vi "Motor Controller two-parameter optimisation.vi"(0 "Settling time (ms)":u32=5000, 1 "Data rate (Hz)":u8(ring)=21 items=["1", "2", "4", "5", "8", "10", "16", "20", "25", "32", "40", "50", "64", "80", "100", "125", "160", "200", "250", "320", "400", "500", "625", "800", "1000"], 2 "N samples":i32=5000, 3 "Kp_start":dbl=9.999999747378752e-05 format="%#_6f", 4 "Kp_end":dbl=0.002 format="%#_6f", 5 "N_points_Kp":i32=30 min=1, 6 "RPM":sgl=600.0 format="%#_6f", 7 "Ti_start (s)":dbl=0.005 format="%#_6f", 8 "COM port":refnum<visa-resource-name>, 9 "Ti_end (s)":dbl=1.0 format="%#_6f", 11 "N_points_Ti":i32=30 min=1) -> (10 "Frm errs":u32, 12 "Chk errs":u32, 14 "Kp (/rpm)":string, 15 "Ti (s)":string, 16 "RPM std. dev. (/min)":string, 17 "Im mean (A)":string, 18 "Im std. dev. (A)":string, 19 "Error out":errorcluster)   [LabVIEW 2020]
uses:
  <vilib>/Math Plots/3D Math Plots/3D Surface/3D Surface XCtrl/3D Surface.xctl
  ctls/CTRL_PID_params.ctl
  <vilib>/Math Plots/3D Math Plots/3D Surface/3D Surface Datatype/Public/Plot Helper (Vector).vi
  <vilib>/Analysis/NI_AALBase.lvlib
  <vilib>/Math Plots/3D Math Plots/3D Surface/3D Surface Datatype/3D Surface Datatype.lvclass
panel:
  out "Ti loop":i32
  out "Kp loop":i32
  in  "Format string":string="%.6e"
  out "Stats plots":refnum<class "3D Plot Datatype.lvclass">[](xcontrol)
  in  "Stop":bool
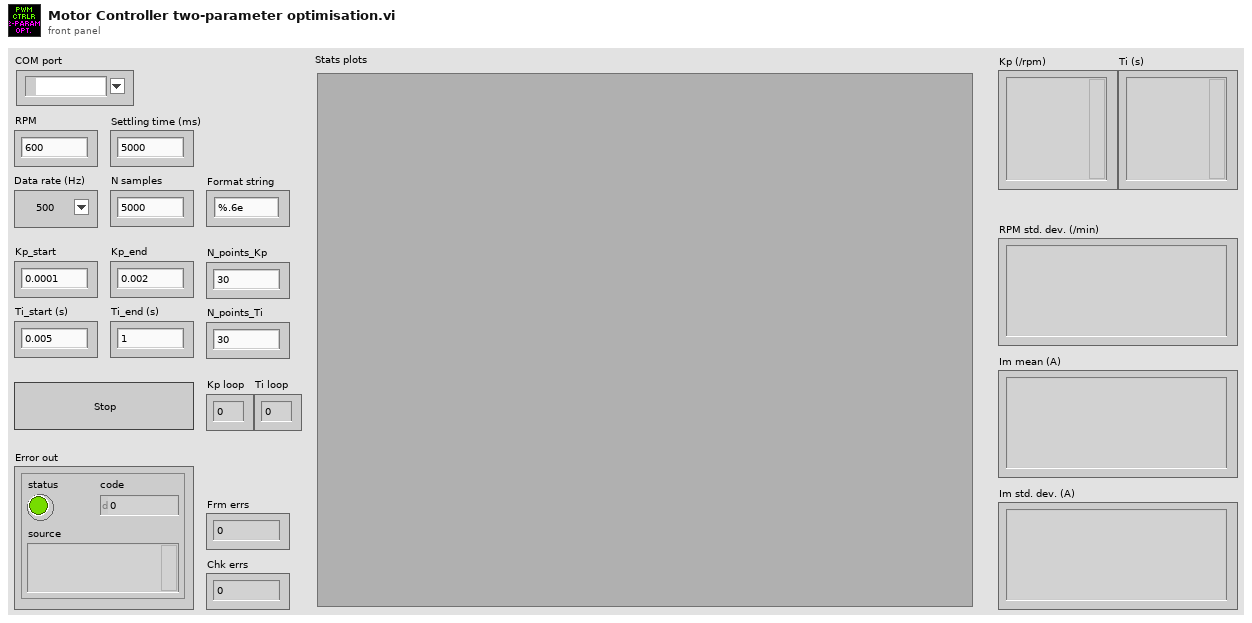
[diagram p1: front panel]
types:
  T1 = typedef "CTRL_EEPROM.ctl" = cluster{"N bits":u8, "dt (s)":sgl, "Kp (/rpm)":sgl, "Ti (s)":sgl, "Td (s)":sgl, "N bits_soft":u8, "dt_soft (s)":sgl, "Kp_soft (/rpm)":sgl, "Ti_soft (s)":sgl, "Td_soft (s)":sgl, "Encoder counting edges":u8, "Encoder PPR":u16, "Final drive ratio (X:1)":sgl, "Current zero offset (A)":sgl, "RS-485 address":u8, "RS-485 baud rate":u32, "Data output period (us)":u32, "RPM setpoint":sgl, "USB streaming enabled":bool, "Operating mode":u8, "Running mode":u8, "EEPROM CRC-16":u16}
  T2 = typedef "CTRL_PID_params.ctl" = cluster{"N bits":u8, "dt (s)":sgl, "Kp (/rpm)":sgl, "Ti (s)":sgl, "Td (s)":sgl}
  T3 = typedef "CTRL_Data_Out.ctl" = cluster{"RPM (/min)":sgl, "I_motor (A)":sgl, "V_photo (V)":sgl, "Duty (-1...1)":sgl}
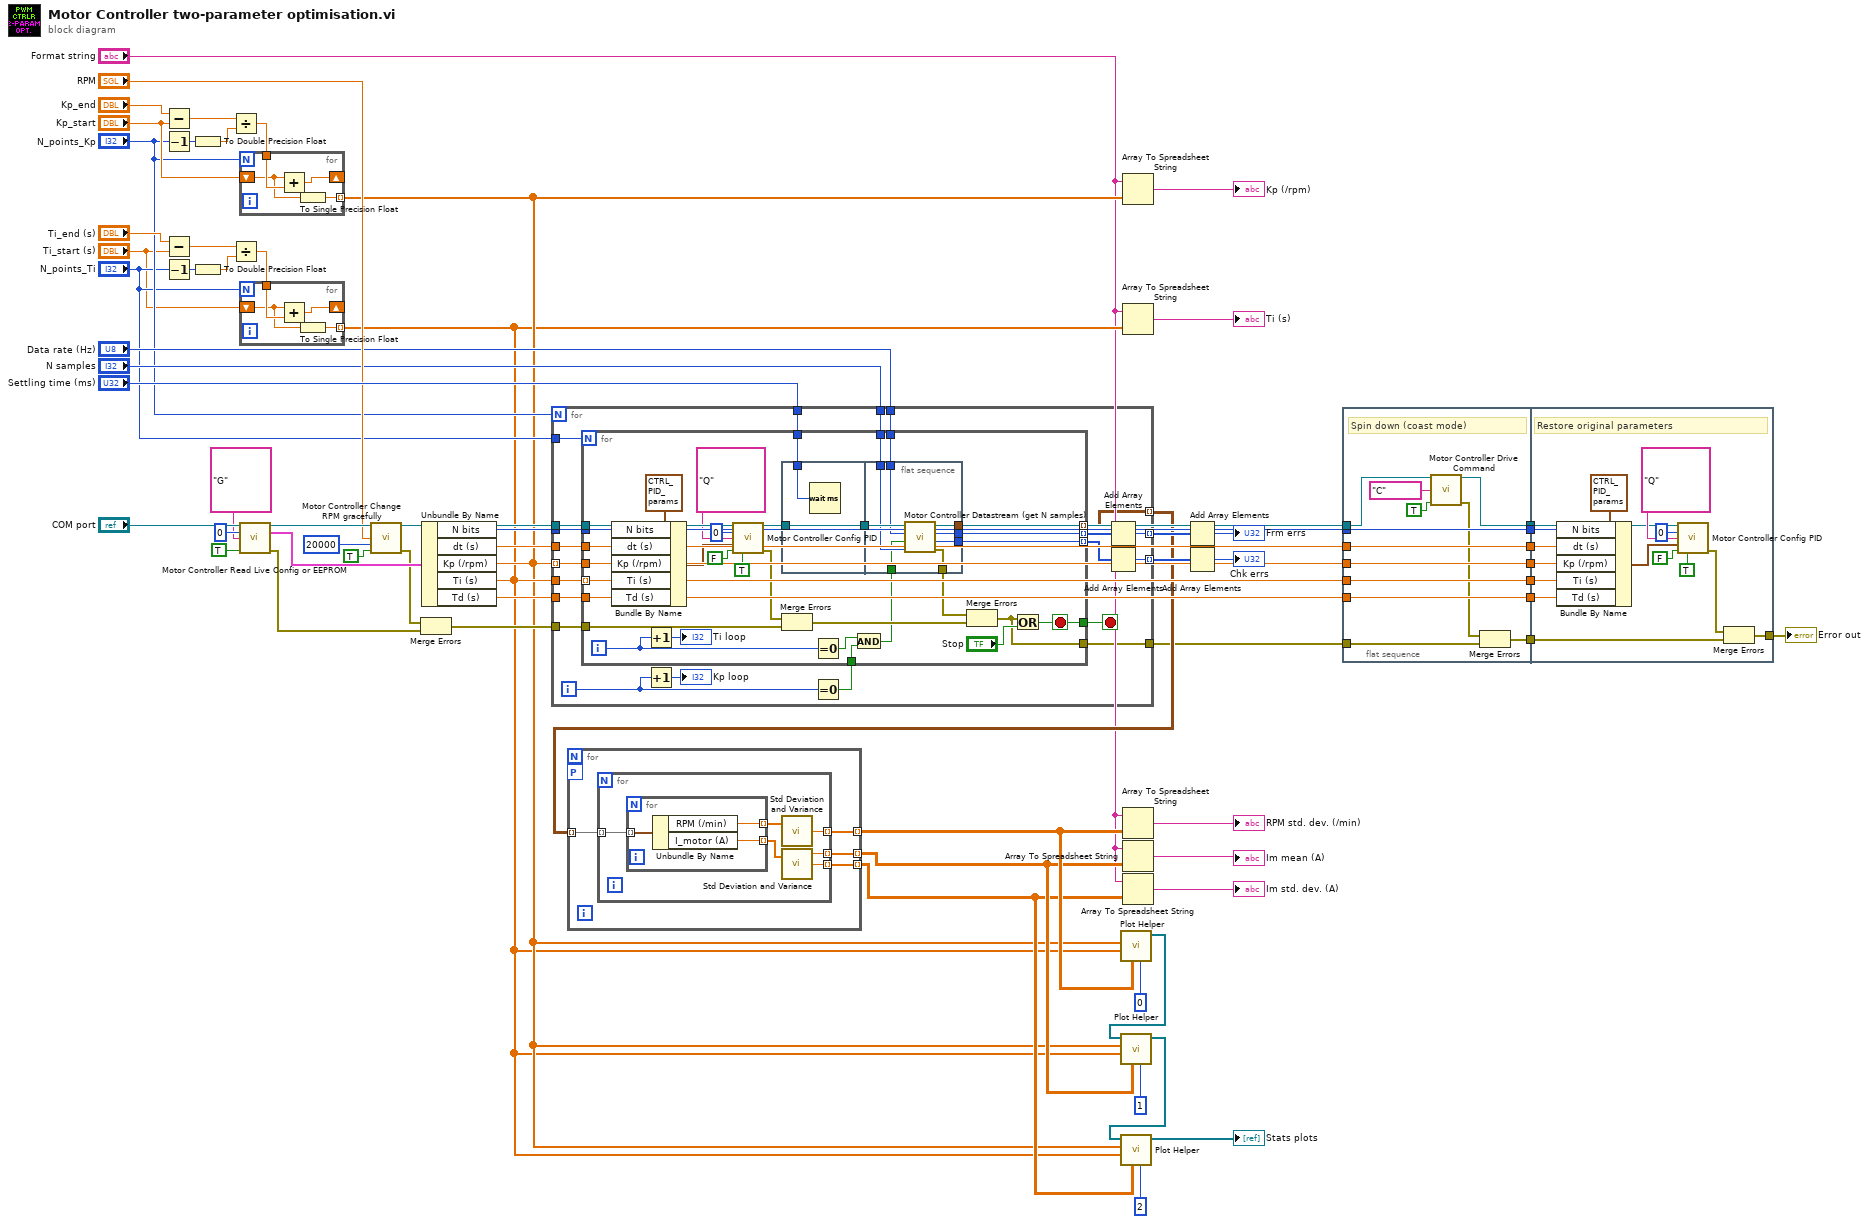
[diagram p0: block diagram]
diagram:
  n1 = Subtract(x="Kp_end", y="Kp_start") -> (x-y=w58:dbl)
  n2 = Decrement(x="N_points_Kp") -> (x-1=w57:i32)
  n3 = Subtract(x="Ti_end (s)", y="Ti_start (s)") -> (x-y=w53:dbl)
  n4 = Decrement(x="N_points_Ti") -> (x-1=w54:i32)
  n5 = To Double Precision Float(number=w57) -> (double precision float=w56:dbl)
  n6 = To Double Precision Float(number=w54) -> (double precision float=w55:dbl)
  n7 = Divide(x=w58, y=w56) -> (x/y=w37:dbl)
  n8 = Divide(x=w53, y=w55) -> (x/y=w34:dbl)
  n9 = for {
    N: "N_points_Kp" -> [_]
    tunnel: w37 -> [w70]
    tunnel: [w68] -> w14 mode=indexing
    shift-right: [w67] -> _
    shift-left: "Kp_start" -> [w69]
    n10 = Add(x=w69, y=w70) -> (x+y=w67:dbl)
    n11 = To Single Precision Float(number=w69) -> (single precision float=w68:sgl)
  }
  n12 = for {
    N: "N_points_Ti" -> [_]
    tunnel: w34 -> [w74]
    tunnel: [w72] -> w13 mode=indexing
    shift-right: [w71] -> _
    shift-left: "Ti_start (s)" -> [w73]
    n13 = Add(x=w73, y=w74) -> (x+y=w71:dbl)
    n14 = To Single Precision Float(number=w73) -> (single precision float=w72:sgl)
  }
  n15 = call "Motor Controller Read Live Config or EEPROM.vi"("COM port"="COM port", "RS-485 addr."=u8 0, "Cmd"="G", "Close port after action"=TRUE) -> ("COM port out"=w46:refnum<visa-resource-name>, "EEPROM"=w48:T1, "Error out"=w42:errorcluster)  [unwired: 8 in, 1 out]
  n16 = call "Motor Controller Change RPM gracefully.vi"("COM port"=w46, "RPM setpoint"="RPM", "Settling time (ms)"=u32 20000, "Close port after action"=TRUE) -> ("COM port out"=w66:refnum<visa-resource-name>, "Error out"=w41:errorcluster)  [unwired: 10 in]
  n17 = Merge Errors(w41, w42) -> (w40:errorcluster)
  n18 = Unbundle By Name(w48) -> ("N bits"=w61:u8, "dt (s)"=w62:sgl, "Kp (/rpm)"=w63:sgl, "Ti (s)"=w64:sgl, "Td (s)"=w65:sgl)
  n19 = for {
    N: "N_points_Kp" -> [_]
    tunnel: w61 -> [w95]
    tunnel: w62 -> [w94]
    tunnel: w65 -> [w93]
    tunnel: "Settling time (ms)" -> [w92]
    tunnel: w66 -> [w91]
    tunnel: w40 -> [w90]
    tunnel: "N samples" -> [w89]
    tunnel: "Data rate (Hz)" -> [w88]
    tunnel: "N_points_Ti" -> [w87]
    tunnel: w13 -> [w86]
    tunnel: w14 -> [w85] mode=indexing
    tunnel: [w80] -> w30 mode=indexing
    tunnel: [w79] -> w31 mode=indexing
    tunnel: [w78] -> w27 mode=indexing
    tunnel: [w77] -> w9
    i -> [w75]
    stop <- w83 stop-if-true
    n20 = Increment(x=w75) -> (x+1=→"Kp loop":i32)
    n21 = Equal To 0?(x=w75) -> (x = 0?=w84:bool)
    n22 = for {
      N: w87 -> [_]
      tunnel: w95 -> [w125]
      tunnel: w94 -> [w124]
      tunnel: w93 -> [w123]
      tunnel: w92 -> [w121]
      tunnel: w91 -> [w117]
      tunnel: w90 -> [w115]
      tunnel: w89 -> [w113]
      tunnel: w88 -> [w112]
      tunnel: [w108] -> w78 mode=indexing
      tunnel: [w107] -> w82 mode=indexing
      tunnel: [w106] -> w81 mode=indexing
      tunnel: w86 -> [w105] mode=indexing
      tunnel: w85 -> [w104]
      tunnel: w84 -> [w101]
      tunnel: [w100] -> w83
      tunnel: [w98] -> w77
      i -> [w97]
      stop <- w100 stop-if-true
      n23 = Bundle By Name(cluster=T2 {"N bits"=15, "dt (s)"=0.002, "Kp (/rpm)"=0.001, "Ti (s)"=0.01, "Td (s)"=0.0} ("PVA params"), "N bits"=w125, "dt (s)"=w124, "Kp (/rpm)"=w104, "Ti (s)"=w105, "Td (s)"=w123) -> (w122:T2)
      n24 = Increment(x=w97) -> (x+1=→"Ti loop":i32)
      n25 = call "Motor Controller Config PID.vi"("COM port"=w117, "RS-485 addr."=u8 0, "Cmd"="Q", "PVA params"=w122, "Set as power-on default"=FALSE, "Close port after action"=TRUE) -> ("COM port out"=w110:refnum<visa-resource-name>, "Error out"=w116:errorcluster)  [unwired: 8 in]
      n26 = flat-sequence {
        tunnel: w121 -> [w129]
        tunnel: [w128] -> w127
        tunnel: w110 -> [w128]
        tunnel: w113 -> [w137]
        tunnel: w112 -> [w136]
        tunnel: [w135] -> w111
        tunnel: w127 -> [w134]
        tunnel: [w133] -> w107
        tunnel: [w132] -> w106
        tunnel: [w131] -> w108
        tunnel: w103 -> [w130]
        frame #0 {
          n27 = Wait (ms)(milliseconds to wait=w129) -> ()  [unwired: 1 out]
        }
        frame #1 {
          n28 = call "Motor Controller Datastream (get N samples).vi"("N samples"=w137, "Set data rate?"=w130, "Data rate (Hz)"=w136, "COM port"=w134) -> ("Error out"=w135:errorcluster, "Chk err"=w132:u32, "Frm err"=w133:u32, "Data cluster array"=w131:T3[])  [unwired: 4 in]
        }
      }
      n29 = Merge Errors(w116, w115) -> (w114:errorcluster)
      n30 = Equal To 0?(x=w97) -> (x = 0?=w102:bool)
      n31 = And(x=w102, y=w101) -> (x .and. y?=w103:bool)
      n32 = Merge Errors(w111, w114) -> (w98:errorcluster)
      n33 = Or(x=w98, y="Stop") -> (x .or. y?=w100:bool)
    }
    n34 = Add Array Elements(numeric array=w82) -> (sum=w79:u32)
    n35 = Add Array Elements(numeric array=w81) -> (sum=w80:u32)
  }
  n36 = for {
    tunnel: w27 -> [w141] mode=indexing
    tunnel: [w140] -> w19 mode=indexing
    tunnel: [w139] -> w15 mode=indexing
    tunnel: [w138] -> w21 mode=indexing
    workers-P: _ -> [_]
    n37 = for {
      tunnel: w141 -> [w147] mode=indexing
      tunnel: [w144] -> w140 mode=indexing
      tunnel: [w143] -> w139 mode=indexing
      tunnel: [w142] -> w138 mode=indexing
      n38 = for {
        tunnel: w147 -> [w150] mode=indexing
        tunnel: [w149] -> w146 mode=indexing
        tunnel: [w148] -> w145 mode=indexing
        n39 = Unbundle By Name(w150) -> ("RPM (/min)"=w149:sgl, "I_motor (A)"=w148:sgl)
      }
      n40 = call <vilib>:"Std Deviation and Variance.vi"("X"=w146) -> ("standard deviation"=w142:dbl)  [unwired: 1 in, 2 out]
      n41 = call <vilib>:"Std Deviation and Variance.vi"("X"=w145) -> ("mean"=w144:dbl, "standard deviation"=w143:dbl)  [unwired: 1 in, 1 out]
    }
  }
  n42 = call-poly <vilib>:"Plot Helper.vi"("Plot ID"=0, "z matrix"=w21, "y vector"=w13, "x vector"=w14) -> ("3D Plot lvclass Array out"=w17:refnum<class "3D Plot Datatype.lvclass">[])  [unwired: 2 in, 5 out]
  n43 = call-poly <vilib>:"Plot Helper.vi"("Plot ID"=1, "z matrix"=w19, "y vector"=w13, "x vector"=w14, "3D Plot lvclass Array in"=w17) -> ("3D Plot lvclass Array out"=w12:refnum<class "3D Plot Datatype.lvclass">[])  [unwired: 1 in, 5 out]
  n44 = call-poly <vilib>:"Plot Helper.vi"("Plot ID"=2, "z matrix"=w15, "y vector"=w13, "x vector"=w14, "3D Plot lvclass Array in"=w12) -> ("3D Plot lvclass Array out"=→"Stats plots":refnum<class "3D Plot Datatype.lvclass">[])  [unwired: 1 in, 5 out]
  n45 = Array To Spreadsheet String(array=w14, 3:"Format string") -> (spreadsheet string=→"Kp (/rpm)":string)  [unwired: 1 in]
  n46 = Array To Spreadsheet String(array=w13, 3:"Format string") -> (spreadsheet string=→"Ti (s)":string)  [unwired: 1 in]
  n47 = Array To Spreadsheet String(array=w21, 3:"Format string") -> (spreadsheet string=→"RPM std. dev. (/min)":string)  [unwired: 1 in]
  n48 = Array To Spreadsheet String(array=w19, 3:"Format string") -> (spreadsheet string=→"Im mean (A)":string)  [unwired: 1 in]
  n49 = Array To Spreadsheet String(array=w15, 3:"Format string") -> (spreadsheet string=→"Im std. dev. (A)":string)  [unwired: 1 in]
  n50 = Add Array Elements(numeric array=w31) -> (sum=→"Frm errs":u32)
  n51 = Add Array Elements(numeric array=w30) -> (sum=→"Chk errs":u32)
  n52 = flat-sequence {
    tunnel: w61 -> [w158]
    tunnel: w62 -> [w159]
    tunnel: w63 -> [w160]
    tunnel: w64 -> [w161]
    tunnel: w65 -> [w162]
    tunnel: w66 -> [w157]
    tunnel: w9 -> [w155]
    tunnel: [w154] -> w7
    tunnel: [w156] -> w6
    tunnel: [w162] -> w5
    tunnel: [w161] -> w4
    tunnel: [w160] -> w3
    tunnel: [w159] -> w2
    tunnel: [w158] -> w1
    tunnel: [w163] -> w8
    tunnel: w7 -> [w164]
    tunnel: w6 -> [w171]
    tunnel: w5 -> [w170]
    tunnel: w4 -> [w169]
    tunnel: w3 -> [w168]
    tunnel: w2 -> [w167]
    tunnel: w1 -> [w166]
    frame #0 {
      # "Spin down (coast mode)"
      n53 = call "Motor Controller Drive Command.vi"("COM port"=w157, "Command"="C", "Close port after action"=TRUE) -> ("COM port out"=w156:refnum<visa-resource-name>, "Error out"=w153:errorcluster)  [unwired: 11 in]
      n54 = Merge Errors(w153, w155) -> (w154:errorcluster)
    }
    frame #1 {
      # "Restore original parameters"
      n55 = Bundle By Name(cluster=T2 {"N bits"=15, "dt (s)"=0.002, "Kp (/rpm)"=0.001, "Ti (s)"=0.01, "Td (s)"=0.0} ("PVA params"), "N bits"=w166, "dt (s)"=w167, "Kp (/rpm)"=w168, "Ti (s)"=w169, "Td (s)"=w170) -> (w173:T2)
      n56 = call "Motor Controller Config PID.vi"("COM port"=w171, "RS-485 addr."=u8 0, "Cmd"="Q", "PVA params"=w173, "Set as power-on default"=FALSE, "Close port after action"=TRUE) -> ("Error out"=w165:errorcluster)  [unwired: 8 in, 1 out]
      n57 = Merge Errors(w165, w164) -> (w163:errorcluster)
    }
  }
  "Error out" <- w8
